vi "Save_Converted.vi"(6 "Top level VI Name":string, 8 "Vi's already saved in":string[](array[string]), 9 "Saved Vis paths in":string[](array[string]), 10 "VI to save":string, 11 "vi reference":refnum<vi>) -> (0 "Vi's already saved out":string[](array[string]), 1 "Error IO":errorcluster, 2 "vi references to save":refnum<vi>[](array[refnum]), 3 "Vi's that need saving":string[](array[string]), 4 "Saved Vis paths Out":string[](array[string]))   [LabVIEW 2010]
panel:
  out "VIType":T1(ring)
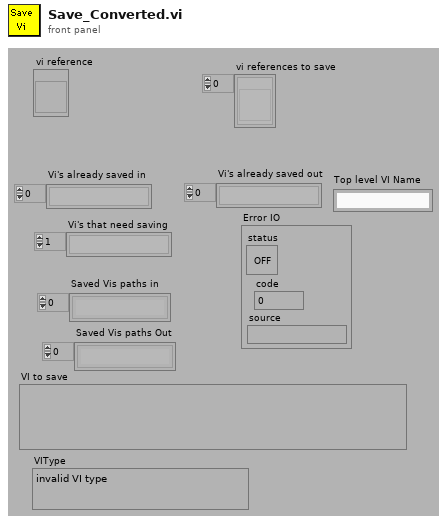
[diagram p1: front panel]
types:
  T1 = enum32{"invalid VI type", "Standard VI", "Control VI", "Global VI"}
  T2 = enum32{"invalid VI type", "Standard VI", "Control VI", "Global VI", "Polymorphic VI", "Configuration VI", "SubSystem", "Facade VI", "Method VI", "Statechart Diagram VI"}
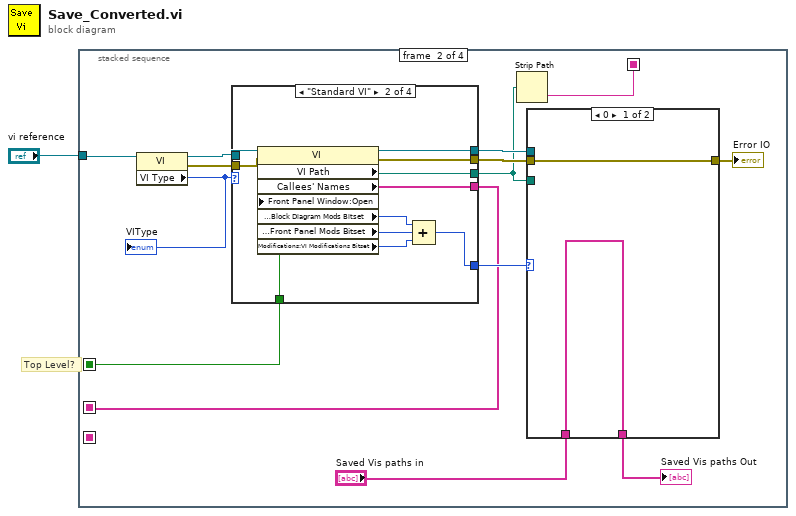
[diagram p0: block diagram]
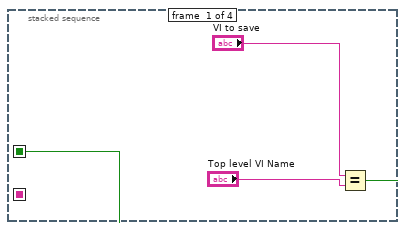
[diagram p2: hidden frame]
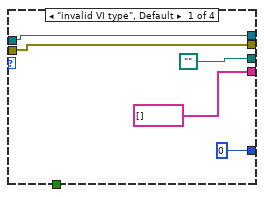
[diagram p3: hidden frame]
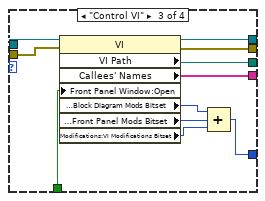
[diagram p4: hidden frame]
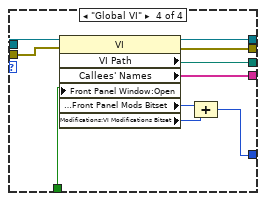
[diagram p5: hidden frame]
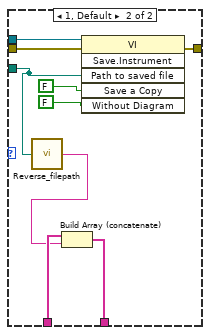
[diagram p6: hidden frame]
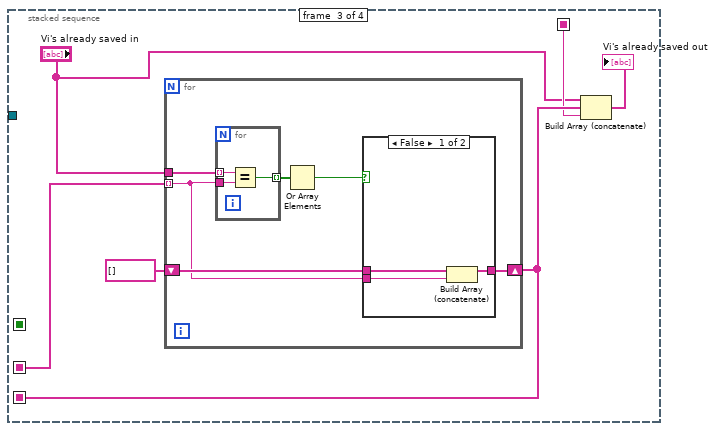
[diagram p7: hidden frame]
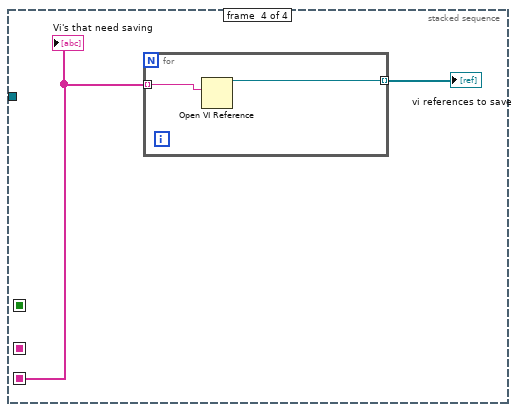
[diagram p9: hidden frame]
diagram:
  # "Top Level?"
  n1 = stacked-sequence {
    seq-local: [_ w12 _ _] -> [_ _ w72 _]
    seq-local: [_ _ w70 _] -> [_ _ _ w87]
    seq-local: [_ w11 _ _] -> [_ _ w68 _]
    seq-local: [w2 _ _ _] -> [_ w5 _ _]
    tunnel: "vi reference" -> [_ w7 _ _]
    frame #0 {
      n2 = Equal?(x="VI to save", y="Top level VI Name") -> (x = y?=w2:bool)
    }
    frame #1 {
      n3 = property class="VI"(reference=w7) -> (reference out=w14:refnum<vi>, error out=w13:errorcluster, "VI Type"=w15:T2)  [unwired: 1 in]
      "VIType" <- w15
      n4 = case shown="\"Standard VI\"" w15 {
        tunnel: [string[] [] ("Callees") w34 w45 w55] -> w12
        tunnel: [path "" ("Path") w33 w44 w54] -> w6
        tunnel: [w21 w32 w43 w53] -> w18
        tunnel: [w22 w31 w42 w52] -> w17
        tunnel: w14 -> [w21 w30 w41 w51]
        tunnel: [u32 0 w24 w37 w47] -> w16
        tunnel: w13 -> [w22 w29 w40 w50]
        tunnel: w5 -> [_ w28 w36 w46]
        frame "invalid VI type", Default {
        }
        frame "Standard VI" {
          n5 = property class="VI"(reference=w30, error in=w29, "Front Panel Window:Open"=w28) -> (reference out=w32:refnum<vi>, error out=w31:errorcluster, "VI Path"=w33:path, "Callees' Names"=w34:string[], "Modifications:Block Diagram Mods Bitset"=w27:u32, "Modifications:Front Panel Mods Bitset"=w26:u32, "Modifications:VI Modifications Bitset"=w25:u32)
          n6 = Compound Arithmetic op=ADD(w27, w26, w25) -> (w24:u32)
        }
        frame "Control VI" {
          n7 = property class="VI"(reference=w41, error in=w40, "Front Panel Window:Open"=w36) -> (reference out=w43:refnum<vi>, error out=w42:errorcluster, "VI Path"=w44:path, "Callees' Names"=w45:string[], "Modifications:Block Diagram Mods Bitset"=w39:u32, "Modifications:Front Panel Mods Bitset"=w38:u32, "Modifications:VI Modifications Bitset"=w35:u32)
          n8 = Compound Arithmetic op=ADD(w39, w38, w35) -> (w37:u32)
        }
        frame "Global VI" {
          n9 = property class="VI"(reference=w51, error in=w50, "Front Panel Window:Open"=w46) -> (reference out=w53:refnum<vi>, error out=w52:errorcluster, "VI Path"=w54:path, "Callees' Names"=w55:string[], "Modifications:Front Panel Mods Bitset"=w49:u32, "Modifications:VI Modifications Bitset"=w48:u32)
          n10 = Compound Arithmetic op=ADD(w49, w48) -> (w47:u32)
        }
      }
      n11 = Strip Path(path=w6) -> (name=w11:string)  [unwired: 1 out]
      n12 = case shown="0" w16 {
        tunnel: w6 -> [_ w59]
        tunnel: w18 -> [_ w64]
        tunnel: w17 -> [w57 w63]
        tunnel: [w57 w62] -> w8
        tunnel: [w56 w60] -> w10
        tunnel: "Saved Vis paths in" -> [w56 w61]
        frame 0 {
        }
        frame 1, Default {
          n13 = call "Reverse_filepath.vi"("Filename"=w59) -> ("Reversed Filepath"=w58:string)
          n14 = Build Array (concatenate)(w61, w58) -> (w60:string[])
          n15 = invoke class="VI" method="Save.Instrument"(reference=w64, error in=w63, "Path to saved file"=w59, "Save a Copy"=FALSE, "Without Diagram"=FALSE) -> (error out=w62:errorcluster)  [unwired: 1 in, 5 out]
        }
      }
      "Error IO" <- w8
      "Saved Vis paths Out" <- w10
    }
    frame #2 {
      n16 = for {
        tunnel: w72 -> [w76] mode=indexing
        tunnel: "Vi's already saved in" -> [w75]
        shift-right: [w77] -> w70
        shift-left: string[] [] -> [w78]
        n17 = for {
          tunnel: w76 -> [w81]
          tunnel: w75 -> [w80] mode=indexing
          tunnel: [w79] -> w74 mode=indexing
          n18 = Equal?(x=w80, y=w81) -> (x = y?=w79:bool)
        }
        n19 = Or Array Elements(Boolean array=w74) -> (logical OR=w73:bool)
        n20 = case shown="False" w73 {
          tunnel: w76 -> [w84 _]
          tunnel: w78 -> [w83 w85]
          tunnel: [w82 w85] -> w77
          frame False {
            n21 = Build Array (concatenate)(w83, w84) -> (w82:string[])
          }
          frame True {
          }
        }
      }
      n22 = Build Array (concatenate)("Vi's already saved in", w70, w68) -> (→"Vi's already saved out":string[])
    }
    frame #3 {
      n23 = for {
        tunnel: w87 -> [w89] mode=indexing
        tunnel: [w88] -> w86 mode=indexing
        n24 = Open VI Reference(vi path=w89) -> (vi reference=w88:refnum<vi>)  [unwired: 1 in, 5 out]
      }
      "vi references to save" <- w86
      "Vi's that need saving" <- w87
    }
  }
